vi "Custom Device CORE.vi"(8 "error in (no error)":errorcluster, 11 "CDW_MetaDataObj":refnum<class "NIVS_Consolidated_CDW_MetaDataObj.lvclass">) -> (0 "error out":errorcluster)   [LabVIEW 2019, in "NIVS_Consolidated_CDW_MetaDataObj.lvclass"]
doc: "This VI is the Core VI for the Custom Device Wizard.\n\nWritten by:\nStephan Daunke\n\nDate:\n2014/01/27\n\nCompany:\nNational Instruments Germany GmbH"
uses:
  NIVS_Consolidated_CDW_MetaDataObj.lvclass
  Action.ctl
  CD Shared lvlib.vi
  CD Shared lvlib.ctl
  CD System Explorer lvlib.vi
  CD System Explorer lvlib.ctl
  Common.ctl
  Utility folder.vi
  Utility folder.ctl
  CD Engine lvlib.vi
  CD Engine lvlib.ctl
  Common.vi
  Add Item - Type.ctl
  Build Spec System Explorer.ctl
  Build Spec Engine.vi
  Build Spec Engine.ctl
  <vilib>/Utility/config.llb/NI_LVConfig.lvlib
  <vilib>/Utility/config.llb/Write Key (String).vi
  <vilib>/Utility/traverseref.llb/TRef TravTarget.ctl
  <vilib>/Utility/Data Type/NI_Data Type.lvlib
  Internal data.ctl
  Template Classes/NIVS_CD Template/NIVS_CD Template.lvclass
  Template Classes/NIVS_PPLCD Template/NIVS_PPLCD Template.lvclass
  Build Spec System Explorer.vi
  <vilib>/Utility/config.llb/Write Key (Path).vi
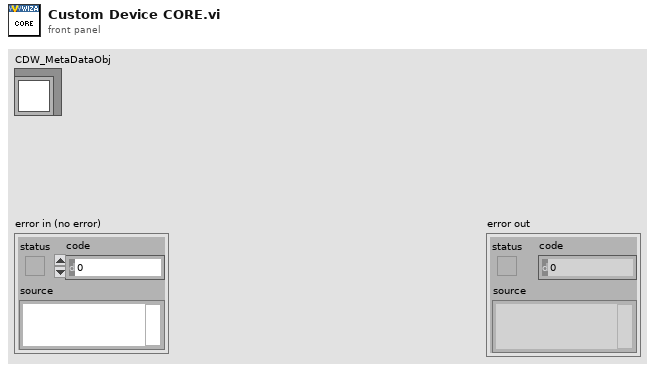
[diagram p1: front panel]
types:
  T1 = typedef "NIVS_Consolidated_CDW_MetaDataObj.lvclass/Internal data.ctl" = cluster{"CD GUID":string, "Extra Page GUIDs":string[], "System Explorer Library":refnum<vi>, "Shared Library":refnum<vi>, "Engine Library":refnum<vi>}
  T2 = typedef "NIVS_Consolidated_CDW_MetaDataObj.lvclass/Action.ctl" = enum16{"Project - Create Custom Device folder", "PC - Create GUID for each extra page", "PC-Utility - Create folder and copy -Copy .LLB to NI VeriStand dir-", "PC-Utility - Change -Copy .LLB to NI VeriStand dir-", "PC-Shared - Create folder and copy Constants.vi", "PC-Shared - Change Constants.vi content", "PC-Shared - Create library", "PC-Shared - Add folders and VIs to library", "PC-System Explorer - Create folder and copy templates", "PC-System Explorer - Create extra pages", "PC-System Explorer - Create library", "PC-System Explorer - Add folders and VIs to library", "PC-Engine - Create folder and copy the RT Template", "PC-Engine - Create library", "PC-Engine - Add virtual folders and VIs to library", "PC-XML - Create and change file", "PC-Help - Copy HTML Files", "Project - Read project file content", "Project - Edit Utility section", "Project - Edit XML section", "Project - Edit Engine Library section", "Project - Edit Shared Library section", "Project - Edit System Explorer Library section", "Project - Edit Custom Device Name", "Project - Edit System Explorer LLB Name", "Project - Edit Engine LLB OS dependent file name", "Project - Copy Configuration file", "Project - Write new project file"}
  T3 = typedef "NIVS_Consolidated_CDW_MetaDataObj.lvclass/Utility folder.ctl" = enum16{"Utility.FolderName", "Utility.PPL Tools Folder Path", "Utility.Copy .llb to NI VeriStand dir.FileName", "Utility.Copy .llb to NI VeriStand dir.FilePathAndName", "Utility.LLB Pre Build.FilePathAndName"}
  T4 = typedef "NIVS_Consolidated_CDW_MetaDataObj.lvclass/CD Shared lvlib.ctl" = enum16{"LibraryFileName", "LibraryFolderName", "ConstantsVI.VIPathAndName", "Shared.FolderName", "Shared.Types.FolderName", "Shared.Constants.VIName", "Shared.Constants.VITemplateName", "Shared.Constants.VITemplatePathAndName", "Shared.CompiledSettings.RelativePath", "Shared.Constants.RelativePath", "Shared.CompiledSettings.Name", "Shared.CompiledSettings.Name.NoExtension", "Shared.CompiledSettings.ClusterName"}
  T5 = typedef "NIVS_Consolidated_CDW_MetaDataObj.lvclass/Common.ctl" = enum16{"ProjectName", "TemplatesFolderName", "PPLTemplatesFolderName", "ProjectTemplatePathAndName", "TimingAndSyncFolderName", "CustomDeviceFolderName", "PathToTemplates", "PathToConfigurationFile", "ProjectConfigurationName"}
  T6 = typedef "NIVS_Consolidated_CDW_MetaDataObj.lvclass/Add Item - Type.ctl" = string
  T7 = typedef "NIVS_Consolidated_CDW_MetaDataObj.lvclass/CD System Explorer lvlib.ctl" = enum16{"LibraryFileName", "LibraryFolderName", "System Explorer.FolderName", "System Explorer.Dynamically Called.FolderName", "System Explorer.Dynamically Called.Extra Pages.FolderName", "System Explorer.Dynamically Called.Extra Pages.TemplatePathAndName", "System Explorer.Dynamically Called.Main Page.VIName", "System Explorer.Dynamically Called.Main Page.TemplatePathAndName", "System Explorer.Dynamically Called.Initialization VI.VIName", "System Explorer.Dynamically Called.Initialization VI.TemplatePathAndName", "System Explorer.SubVI.FolderName", "System Explorer.Types.FolderName", "System Explorer.ActionVIOnCompile.VIName", "System Explorer.ExportConfigRTM.VIName", "System Explorer.LoadHelpFile.VIName"}
  T8 = typedef "TRef TravTarget.ctl" = enum16{"FP", "BD", "Other"}
  T9 = typedef "NIVS_Consolidated_CDW_MetaDataObj.lvclass/CD Engine lvlib.ctl" = enum16{"LibraryFileName", "LibraryFolderName", "Engine.FolderName", "Engine.Init.FolderName", "Engine.Run.FolderName", "Engine.Shutdown.FolderName", "Types.FolderName", "Engine.RT Driver VI.TemplatePath", "Engine.RT Driver VI.FileName", "Engine.RTStateVariables.Name", "Engine.RTStateVariables.Name.NoExtension", "Engine.Async.NameExtension", "Engine.Async.TemplateName"}
  T10 = typedef "NIVS_Consolidated_CDW_MetaDataObj.lvclass/Build Spec System Explorer.ctl" = enum16{"Destinations.LLBFileName"}
  T11 = typedef "NIVS_Consolidated_CDW_MetaDataObj.lvclass/Build Spec Engine.ctl" = enum16{"Destinations.LLBWindowsFileName", "Destinations.LLBVxWorksFileName", "Destinations.LLBPharlapFileName", "Destinations.LLBLinuxARMFileName", "Destinations.LLBLinux64FileName"}
  T12 = enum16{"open", "replace", "create", "open or create", "replace or create", "replace or create with confirmation"}
  T13 = typedef "NI_LVConfig.lvlib/Config Data RefNum.ctl" = refnum<k1>
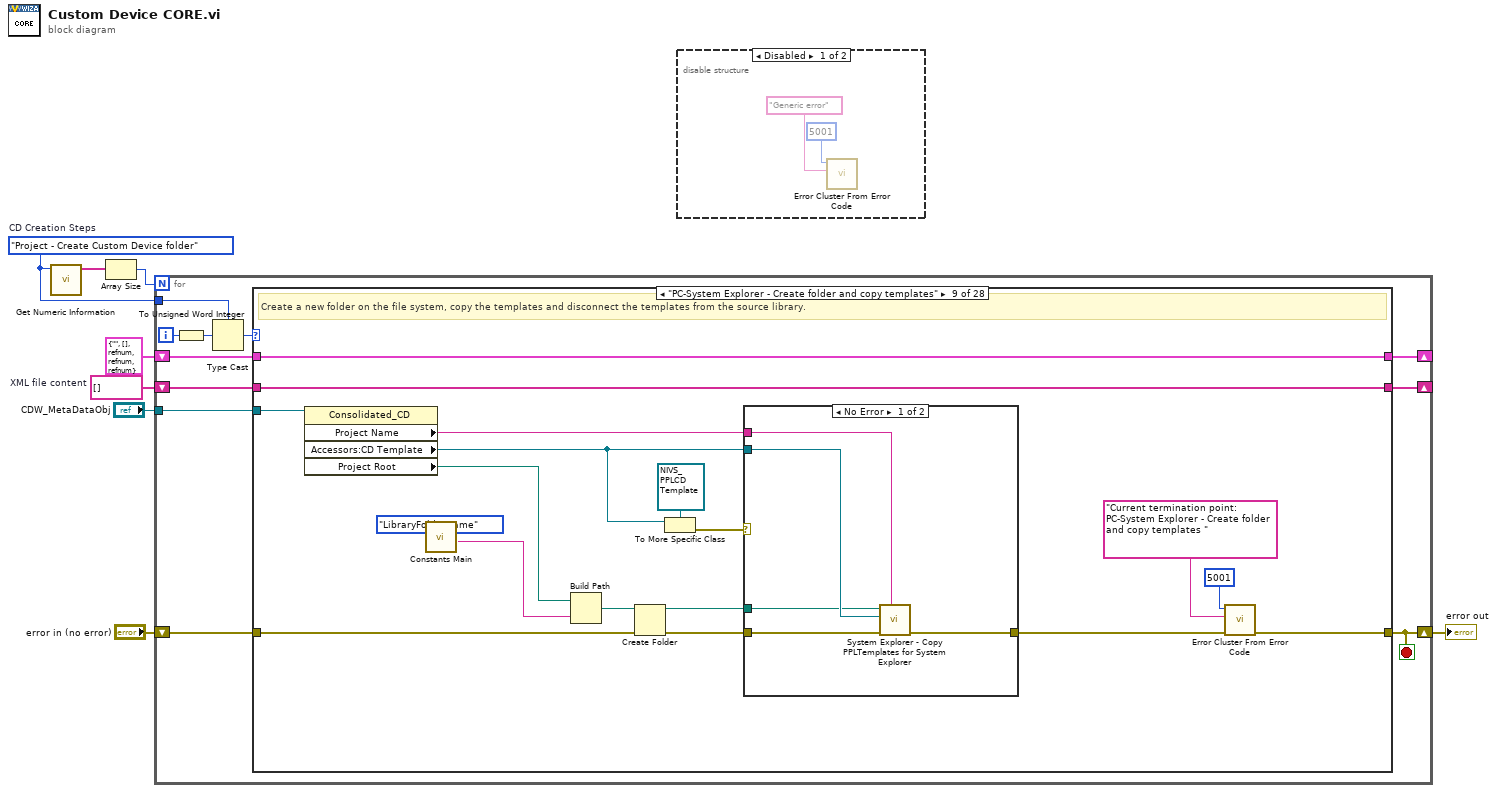
[diagram p0: block diagram]
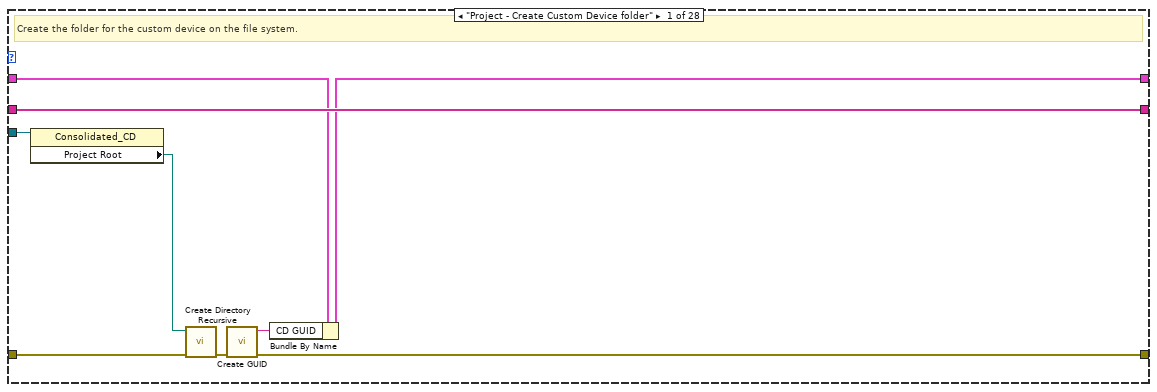
[diagram p3: hidden frame]
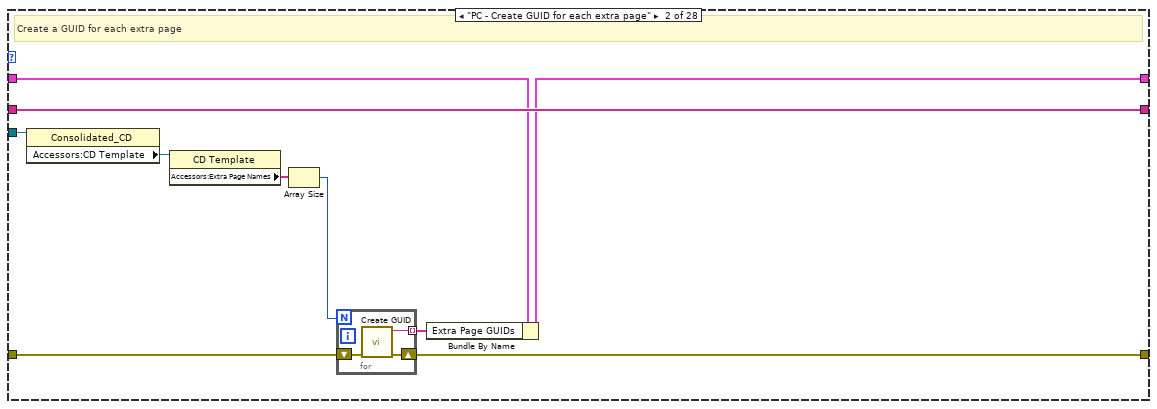
[diagram p4: hidden frame]
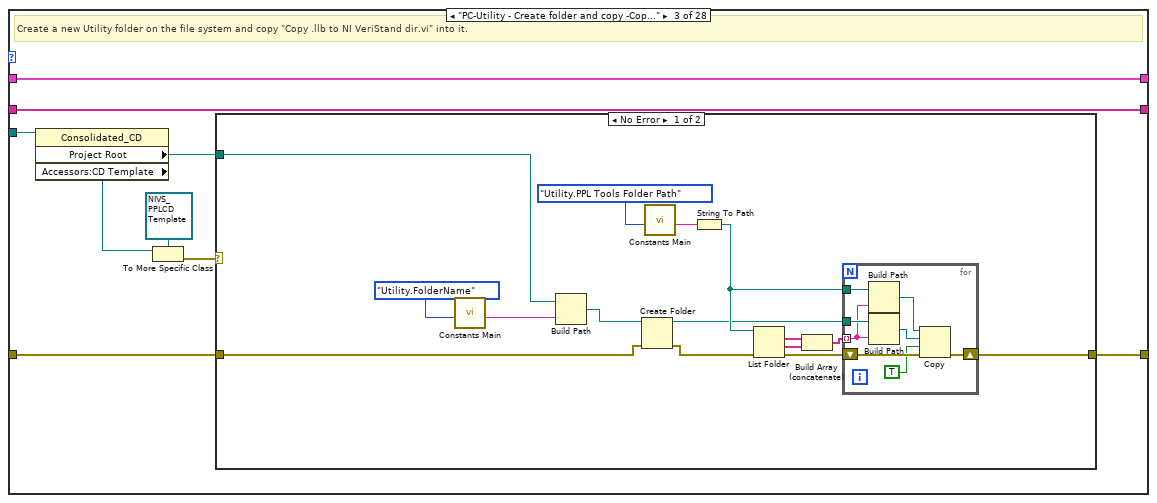
[diagram p5: hidden frame]
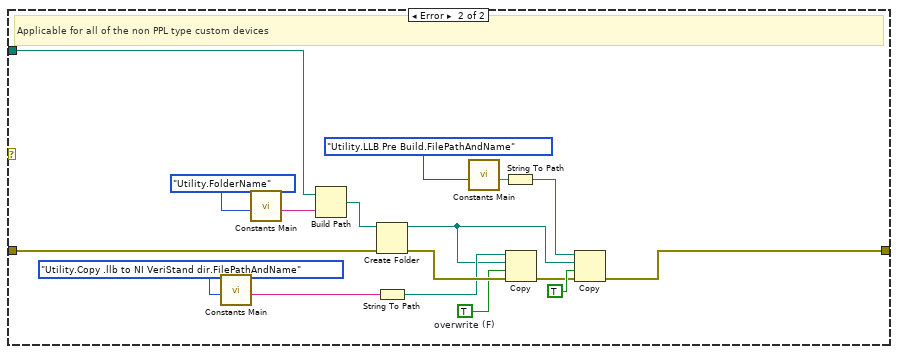
[diagram p6: hidden frame]
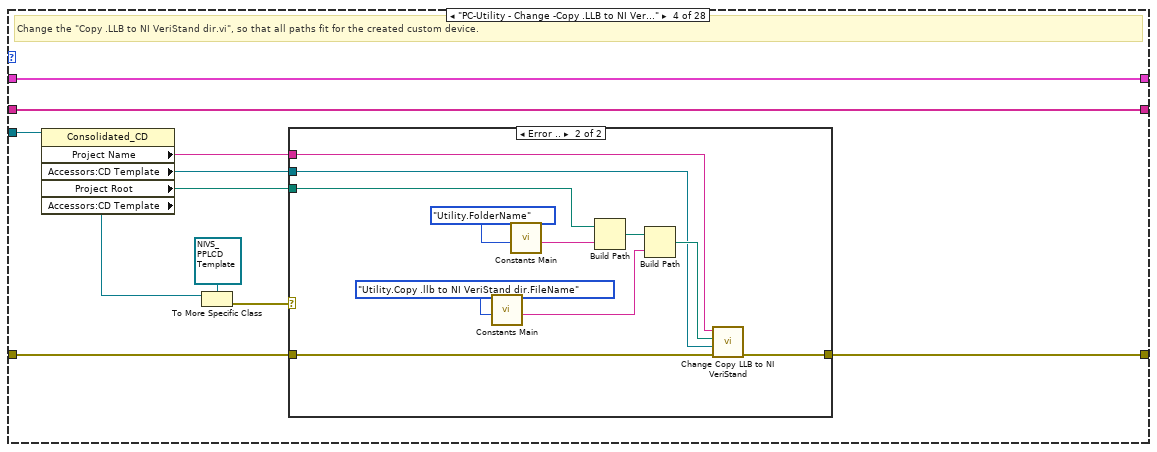
[diagram p7: hidden frame]
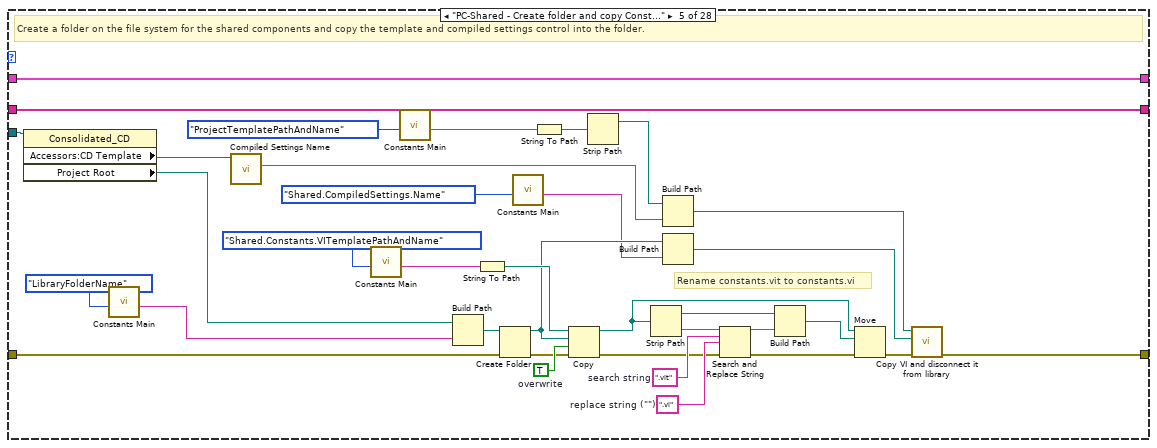
[diagram p9: hidden frame]
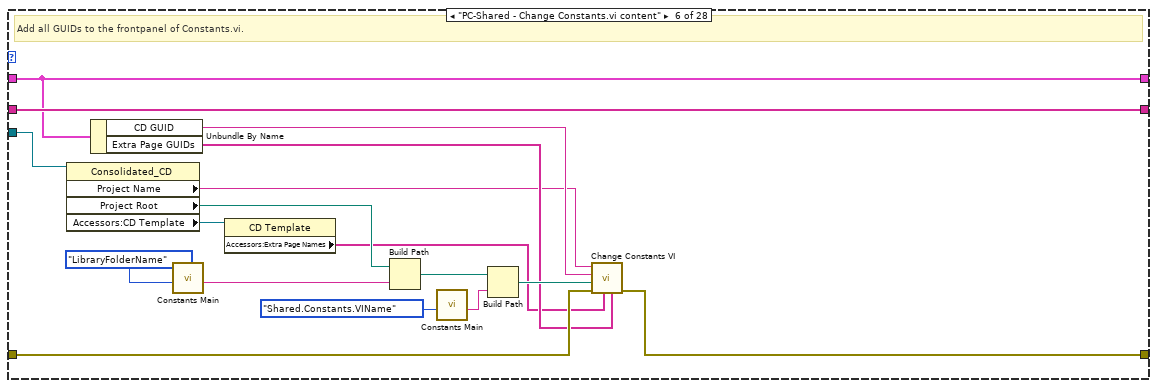
[diagram p10: hidden frame]
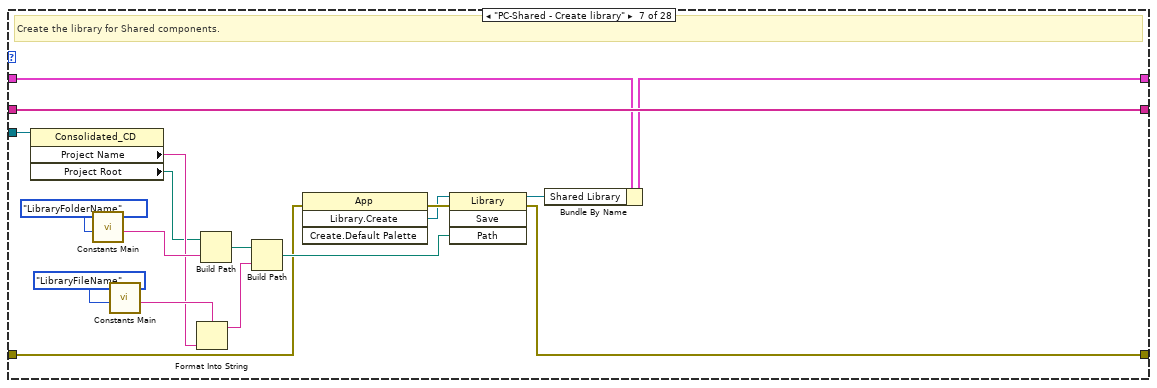
[diagram p11: hidden frame]
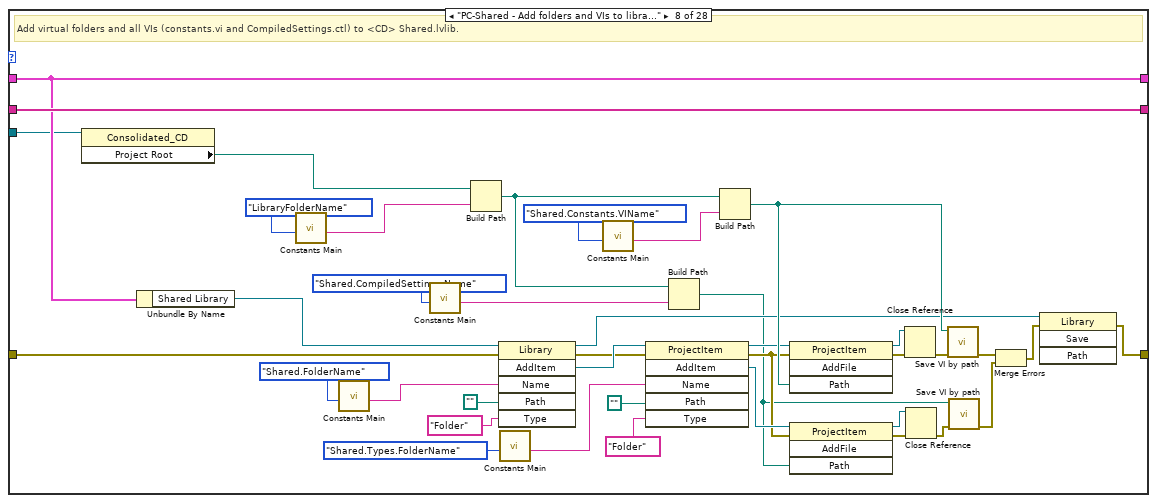
[diagram p12: hidden frame]
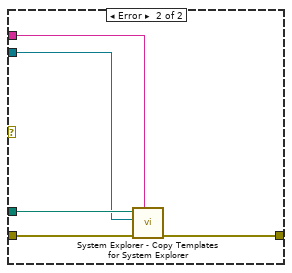
[diagram p13: hidden frame]
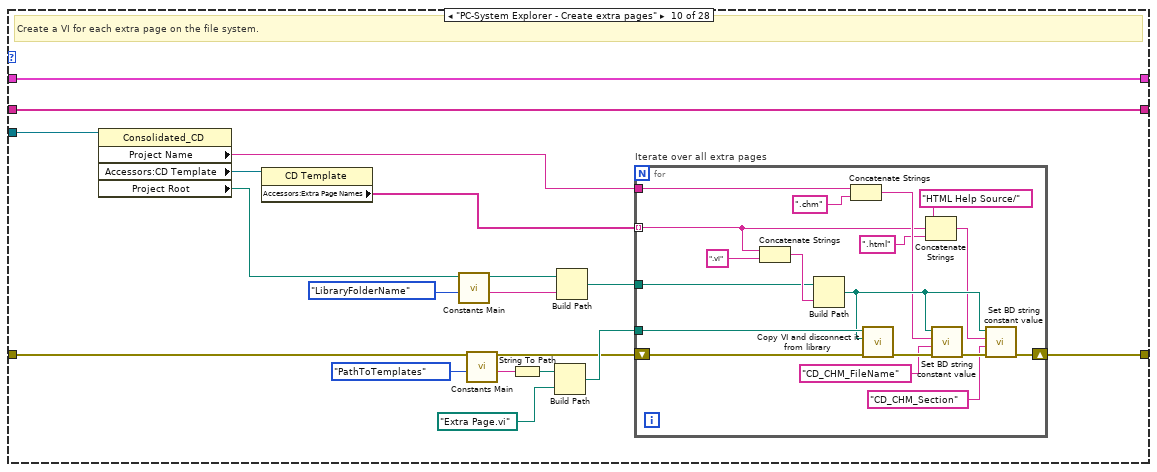
[diagram p14: hidden frame]
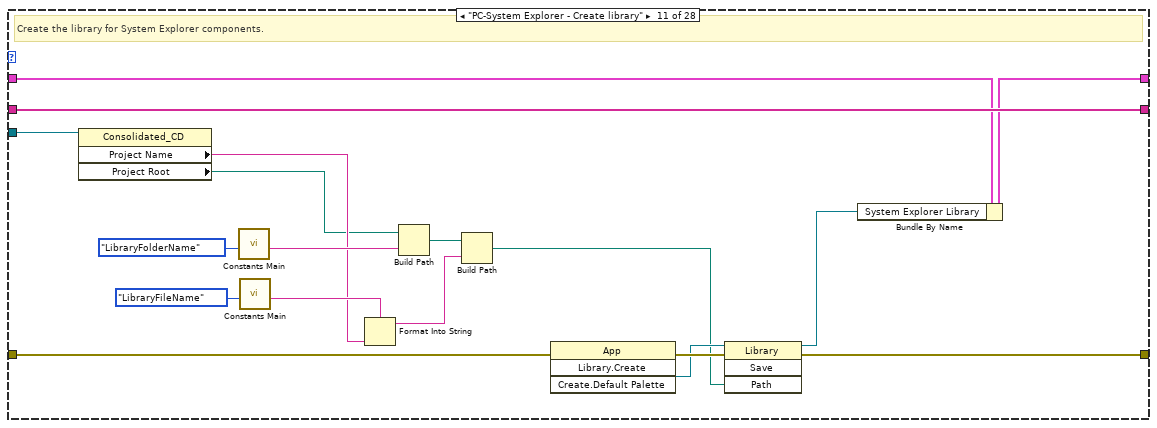
[diagram p15: hidden frame]
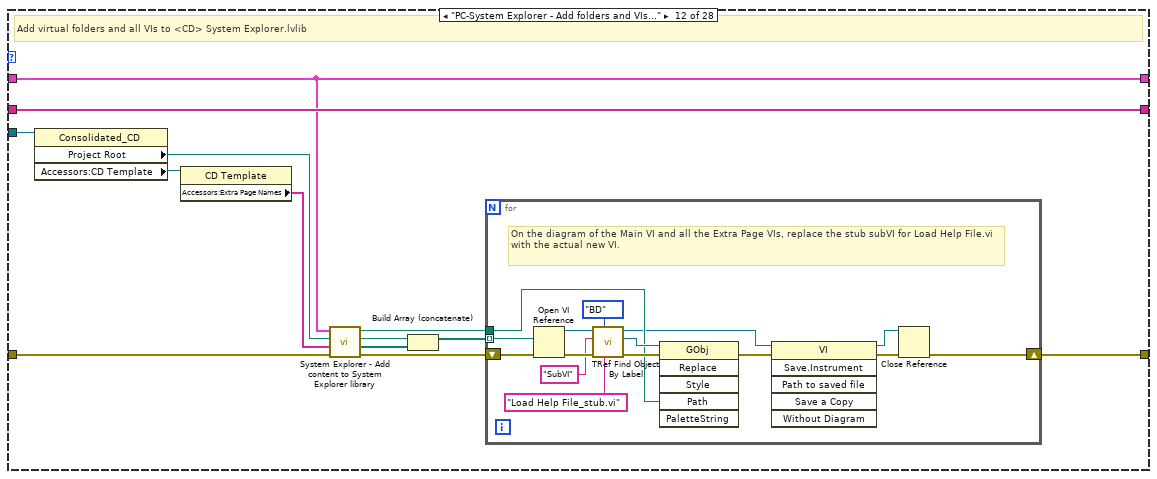
[diagram p16: hidden frame]
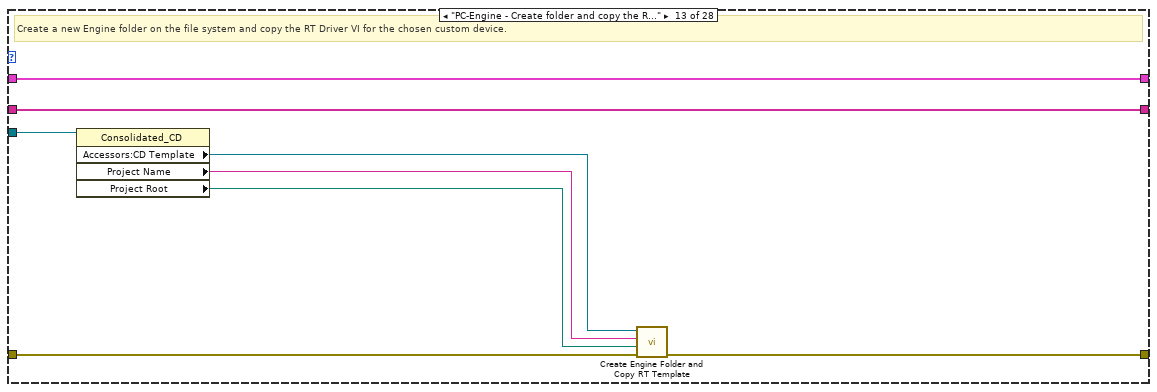
[diagram p17: hidden frame]
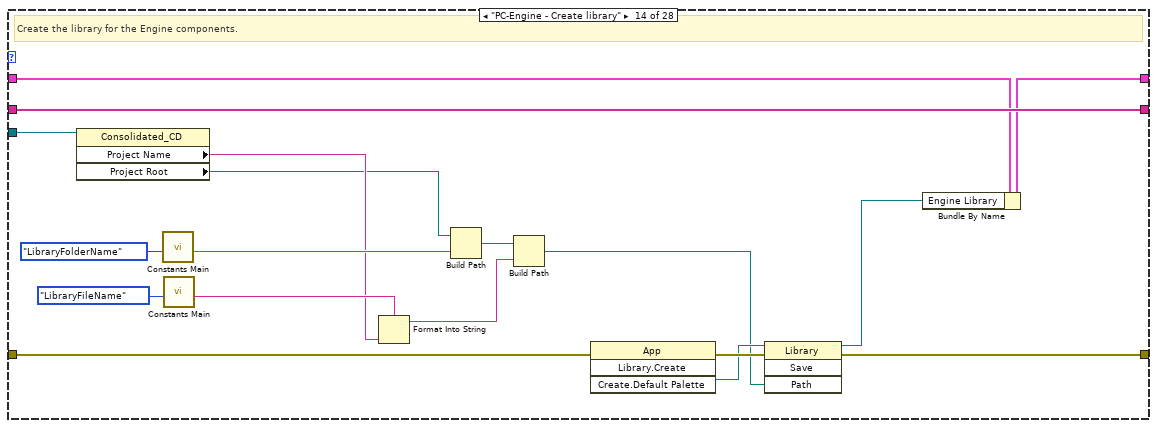
[diagram p18: hidden frame]
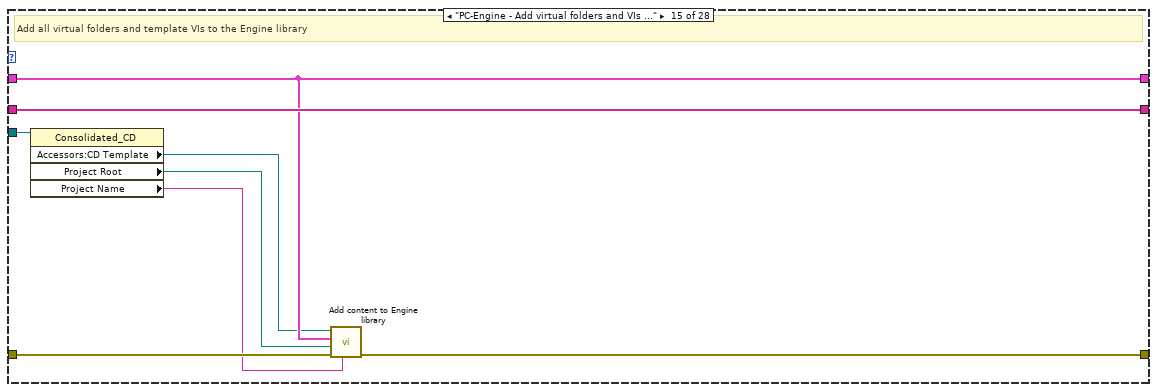
[diagram p19: hidden frame]
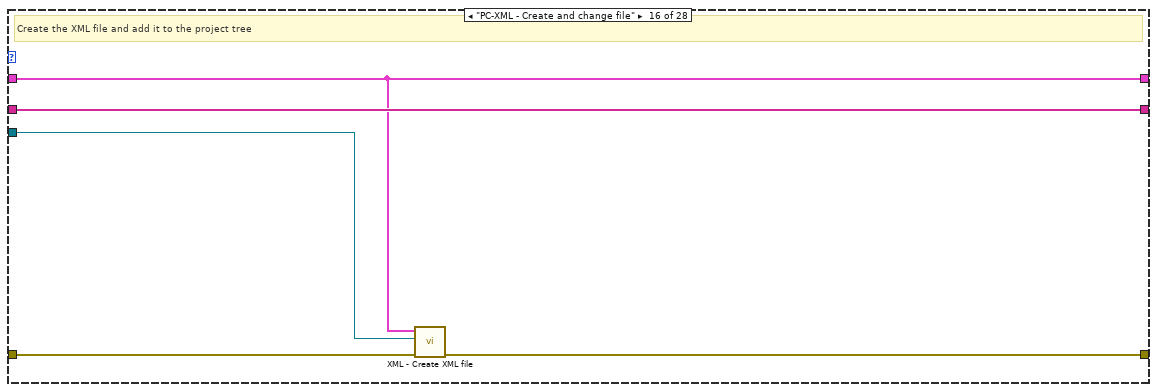
[diagram p20: hidden frame]
diagram:
  w4 = Action."Project - Create Custom Device folder"  # CD Creation Steps
  w5 = string[] []  # XML file content
  n1 = call <vilib>:"Get Numeric Information.vi"("variant"=w4) -> ("enum names"=w3:string[])  [unwired: 7 in, 3 out]
  n2 = Array Size(array=w3) -> (size(s)=w2:i32)
  n3 = for {
    N: w2 -> [_]
    shift-right: [w16] -> _
    shift-left: T1 {"CD GUID"="", "Extra Page GUIDs"=[], "System Explorer Library"=refnum, "Shared Library"=refnum, "Engine Library"=refnum} ("CD Wizard - Internal Data") -> [w18]
    shift-right: [w15] -> _
    shift-left: w5 -> [w17]
    shift-right: [w14] -> w6
    shift-left: "error in (no error)" -> [w19]
    tunnel: w4 -> [w12]
    tunnel: "CDW_MetaDataObj" -> [w11]
    i -> [w13]
    stop <- w14 stop-if-true
    n4 = To Unsigned Word Integer(number=w13) -> (unsigned 16bit integer=w9:u16)
    n5 = Type Cast(type=w12, x=w9) -> (*(type *) &x=w10:T2)
    n6 = case shown="\"PC-System Explorer - Create folder and copy templates\"" w10 {
      tunnel: w19 -> [w24 w37 w46 w96 w118 w158 w169 w186 w231 w256 w289 w315 w338 w343 w364 w369 w387 w417 w430 w462 w481 w485 w515 w549 w560 w578 w615 w631]
      tunnel: [w25 w36 w49 w100 w120 w164 w170 w184 w223 w266 w290 w310 w337 w346 w363 w368 w386 w423 w439 w467 w480 w495 w519 w548 w567 w590 w614 w638] -> w14
      tunnel: w18 -> [w22 w34 w48 w99 w119 w155 w173 w204 w234 w265 w295 w313 w336 w350 w361 w367 w382 w429 w442 w464 w479 w486 w516 w545 w564 w596 w627 w663]
      tunnel: w17 -> [w28 w38 w50 w101 w148 w165 w183 w222 w240 w267 w303 w316 w339 w357 w365 w370 w409 _ w441 w466 w478 w490 w517 w546 w562 w591 w626 w657]
      tunnel: [w27 w33 w48 w99 w119 w155 w172 w204 w234 w265 w296 w313 w336 w349 w361 w367 w382 w429 w442 w464 w479 w486 w516 w545 w564 w596 w627 w663] -> w16
      tunnel: [w28 w38 w50 w101 w148 w165 w183 w222 w240 w267 w303 w316 w339 w357 w365 w370 w409 w422 w440 w465 w482 w496 w518 w547 w561 w579 w626 w657] -> w15
      tunnel: w11 -> [w21 w32 w45 w98 w117 w157 w168 w188 w233 w255 w288 w309 w335 w342 w362 w366 w376 _ _ w461 w477 w484 w514 w544 w559 w577 w620 w630]
      frame "Project - Create Custom Device folder" {
        # "Create the folder for the custom device on the file system."
        n7 = property class="Consolidated_CD"(reference=w21) -> ("Project Root"=w20:path)  [unwired: 1 in, 2 out]
        n8 = call <vilib>:"Create Directory Recursive.vi"("error in (no error)"=w24, "directory"=w20) -> ("error out"=w23:errorcluster)  [unwired: 3 in, 2 out]
        n9 = call "Create GUID.vi"("error in (no error)"=w23) -> ("error out"=w25:errorcluster, "Generated GUID"=w26:string)  [unwired: 9 in]
        n10 = Bundle By Name(cluster=w22, "CD GUID"=w26) -> (w27:T1)
      }
      frame "PC - Create GUID for each extra page" {
        # "Create a GUID for each extra page"
        n11 = property class="Consolidated_CD"(reference=w32) -> ("Accessors:CD Template"=w31:refnum<class "NIVS_CD Template.lvclass">)  [unwired: 1 in, 2 out]
        n12 = property class="CD Template"(reference=w31) -> ("Accessors:Extra Page Names"=w30:string[])  [unwired: 1 in, 2 out]
        n13 = Array Size(array=w30) -> (size(s)=w29:i32)
        n14 = for {
          N: w29 -> [_]
          shift-right: [w40] -> w36
          shift-left: w37 -> [w41]
          tunnel: [w39] -> w35 mode=indexing
          n15 = call "Create GUID.vi"("error in (no error)"=w41) -> ("error out"=w40:errorcluster, "Generated GUID"=w39:string)  [unwired: 9 in]
        }
        n16 = Bundle By Name(cluster=w34, "Extra Page GUIDs"=w35) -> (w33:T1)
      }
      frame "PC-Utility - Create folder and copy -Copy .LLB to NI VeriStand dir-" {
        # "Create a new Utility folder on the file system and copy \"Copy .llb to NI VeriStand dir.vi\" into it."
        n17 = property class="Consolidated_CD"(reference=w45) -> ("Project Root"=w47:path, "Accessors:CD Template"=w42:refnum<class "NIVS_CD Template.lvclass">)  [unwired: 1 in, 2 out]
        n18 = To More Specific Class(target class=refnum<class "NIVS_PPLCD Template.lvclass"> refnum ("NIVS_PPLCD Template.lvclass"), reference=w42) -> (error out=w43:errorcluster)  [unwired: 1 in, 1 out]
        n19 = case shown="No Error" w43 {
          tunnel: [w51 w77] -> w49
          tunnel: w47 -> [w59 w76]
          tunnel: w46 -> [w60 w75]
          frame No Error {
            n20 = call-poly "Constants Main.vi"("Action"=Utility_folder."Utility.FolderName") -> ("Output"=w61:string)  [unwired: 10 in]
            n21 = Build Path(base path=w59, name or relative path=w61) -> (appended path=w65:path)
            n22 = Create Folder(path (use dialog)=w65, error in=w60) -> (created path=w56:path, error out=w55:errorcluster)  [unwired: 1 in, 1 out]
            n23 = call-poly "Constants Main.vi"("Action"=Utility_folder."Utility.PPL Tools Folder Path") -> ("Output"=w63:string)  [unwired: 10 in]
            n24 = String To Path(string=w63) -> (path=w57:path)
            n25 = List Folder(path=w57, error in=w55) -> (filenames=w54:string[], folder names=w53:string[], error out=w58:errorcluster)  [unwired: 2 in, 1 out]
            n26 = Build Array (concatenate)(w54, w53) -> (w52:string[])
            n27 = for {
              tunnel: w52 -> [w68] mode=indexing
              tunnel: w57 -> [w71]
              shift-right: [w72] -> w51
              shift-left: w58 -> [w73]
              tunnel: w56 -> [w69]
              n28 = Build Path(base path=w71, name or relative path=w68) -> (appended path=w70:path)
              n29 = Build Path(base path=w69, name or relative path=w68) -> (appended path=w67:path)
              n30 = Copy(8:w73, 9:TRUE ("overwrite (F)"), 10:w67, 11:w70) -> (0:w72:errorcluster)  [unwired: 1 in, 2 out]
            }
          }
          frame Error {
            w88 = TRUE  # overwrite (F)
            # "Applicable for all of the non PPL type custom devices"
            n31 = call-poly "Constants Main.vi"("Action"=Utility_folder."Utility.Copy .llb to NI VeriStand dir.FilePathAndName") -> ("Output"=w86:string)  [unwired: 10 in]
            n32 = call-poly "Constants Main.vi"("Action"=Utility_folder."Utility.FolderName") -> ("Output"=w83:string)  [unwired: 10 in]
            n33 = Build Path(base path=w76, name or relative path=w83) -> (appended path=w90:path)
            n34 = Create Folder(path (use dialog)=w90, error in=w75) -> (created path=w82:path, error out=w89:errorcluster)  [unwired: 1 in, 1 out]
            n35 = String To Path(string=w86) -> (path=w85:path)
            n36 = call-poly "Constants Main.vi"("Action"=Utility_folder."Utility.LLB Pre Build.FilePathAndName") -> ("Output"=w80:string)  [unwired: 10 in]
            n37 = String To Path(string=w80) -> (path=w79:path)
            n38 = Copy(8:w89, 9:w88, 10:w82, 11:w85) -> (0:w74:errorcluster)  [unwired: 3 out]
            n39 = Copy(8:w74, 9:TRUE ("overwrite (F)"), 10:w82, 11:w79) -> (0:w77:errorcluster)  [unwired: 3 out]
          }
        }
      }
      frame "PC-Utility - Change -Copy .LLB to NI VeriStand dir-" {
        # "Change the \"Copy .LLB to NI VeriStand dir.vi\", so that all paths fit for the created custom device."
        n40 = property class="Consolidated_CD"(reference=w98) -> ("Project Name"=w97:string, "Accessors:CD Template"=w93:refnum<class "NIVS_CD Template.lvclass">, "Project Root"=w95:path, "Accessors:CD Template"=w92:refnum<class "NIVS_CD Template.lvclass">)  [unwired: 1 in, 2 out]
        n41 = To More Specific Class(target class=refnum<class "NIVS_PPLCD Template.lvclass"> refnum ("NIVS_PPLCD Template.lvclass"), reference=w92) -> (error out=w91:errorcluster)  [unwired: 1 in, 1 out]
        n42 = case shown="Error .." w91 {
          tunnel: [w102 w108] -> w100
          tunnel: w97 -> [_ w106]
          tunnel: w96 -> [w102 w105]
          tunnel: w95 -> [_ w104]
          tunnel: w93 -> [_ w103]
          frame No Error {
            # "No need to do this for the PPL based CDs"
          }
          frame Error {
            n43 = call-poly "Constants Main.vi"("Action"=Utility_folder."Utility.Copy .llb to NI VeriStand dir.FileName") -> ("Output"=w109:string)  [unwired: 10 in]
            n44 = call-poly "Constants Main.vi"("Action"=Utility_folder."Utility.FolderName") -> ("Output"=w111:string)  [unwired: 10 in]
            n45 = Build Path(base path=w104, name or relative path=w111) -> (appended path=w110:path)
            n46 = Build Path(base path=w110, name or relative path=w109) -> (appended path=w107:path)
            n47 = call "Change Copy LLB to NI VeriStand.vi"("error in (no error)"=w105, "CD Template"=w103, "Copy .LLB to ... path"=w107, "CD Name"=w106) -> ("error out"=w108:errorcluster)  [unwired: 7 in]
          }
        }
      }
      frame "PC-Shared - Create folder and copy Constants.vi" {
        w137 = ".vi"  # replace string ("")
        w138 = ".vit"  # search string
        w142 = TRUE  # overwrite
        # "Rename constants.vit to constants.vi"
        # "Create a folder on the file system for the shared components and copy the template and compiled settings control into the folder."
        n48 = property class="Consolidated_CD"(reference=w117) -> ("Accessors:CD Template"=w115:refnum<class "NIVS_CD Template.lvclass">, "Project Root"=w116:path)  [unwired: 1 in, 2 out]
        n49 = call-poly "Constants Main.vi"("Action"=CD_Shared_lvlib."LibraryFolderName") -> ("Output"=w145:string)  [unwired: 10 in]
        n50 = call-dynamic "Compiled Settings Name.vi"("CD Template in"=w115) -> ("Compiled Settings Name"=w114:string)  [unwired: 10 in]
        n51 = call-poly "Constants Main.vi"("Action"=CD_Shared_lvlib."Shared.Constants.VITemplatePathAndName") -> ("Output"=w143:string)  [unwired: 10 in]
        n52 = call-poly "Constants Main.vi"("Action"=Common."ProjectTemplatePathAndName") -> ("Output"=w129:string)  [unwired: 10 in]
        n53 = Build Path(base path=w116, name or relative path=w145) -> (appended path=w147:path)
        n54 = String To Path(string=w143) -> (path=w135:path)
        n55 = Create Folder(path (use dialog)=w147, error in=w118) -> (created path=w126:path, error out=w136:errorcluster)  [unwired: 1 in, 1 out]
        n56 = call-poly "Constants Main.vi"("Action"=CD_Shared_lvlib."Shared.CompiledSettings.Name") -> ("Output"=w121:string)  [unwired: 10 in]
        n57 = String To Path(string=w129) -> (path=w128:path)
        n58 = Copy(8:w136, 9:w142, 10:w126, 11:w135) -> (0:w134:errorcluster, 3:w131:path)  [unwired: 2 out]
        n59 = Strip Path(path=w128) -> (stripped path=w127:path)  [unwired: 1 out]
        n60 = Strip Path(path=w131) -> (stripped path=w141:path, name=w140:string)
        n61 = Build Path(base path=w127, name or relative path=w114) -> (appended path=w125:path)
        n62 = Build Path(base path=w126, name or relative path=w121) -> (appended path=w124:path)
        n63 = Search and Replace String(input string=w140, search string=w138, replace string=w137, error in=w134) -> (result string=w139:string, error out=w133:errorcluster)  [unwired: 4 in, 2 out]
        n64 = Build Path(base path=w141, name or relative path=w139) -> (appended path=w132:path)
        n65 = Move(source path=w131, error in=w133, 10:w132) -> (error out=w123:errorcluster)  [unwired: 2 in, 2 out]
        n66 = call "Copy VI and disconnect it from library.vi"("error in (no error)"=w123, "VI Target Path"=w124, "VI Source Path"=w125) -> ("error out"=w120:errorcluster)  [unwired: 8 in]
      }
      frame "PC-Shared - Change Constants.vi content" {
        # "Add all GUIDs to the frontpanel of Constants.vi."
        n67 = property class="Consolidated_CD"(reference=w157) -> ("Project Name"=w151:string, "Project Root"=w156:path, "Accessors:CD Template"=w150:refnum<class "NIVS_CD Template.lvclass">)  [unwired: 1 in, 2 out]
        n68 = Unbundle By Name(w155) -> ("CD GUID"=w153:string, "Extra Page GUIDs"=w152:string[])
        n69 = call-poly "Constants Main.vi"("Action"=CD_Shared_lvlib."LibraryFolderName") -> ("Output"=w159:string)  [unwired: 10 in]
        n70 = property class="CD Template"(reference=w150) -> ("Accessors:Extra Page Names"=w149:string[])  [unwired: 1 in, 2 out]
        n71 = Build Path(base path=w156, name or relative path=w159) -> (appended path=w163:path)
        n72 = call-poly "Constants Main.vi"("Action"=CD_Shared_lvlib."Shared.Constants.VIName") -> ("Output"=w161:string)  [unwired: 10 in]
        n73 = Build Path(base path=w163, name or relative path=w161) -> (appended path=w154:path)
        n74 = call "Change Constants VI.vi"("Extra Page GUIDs"=w152, "Extra Page Names"=w149, "error in (no error)"=w158, "Constants.vi path"=w154, "CD GUID"=w153, "CD Name"=w151) -> ("error out"=w164:errorcluster)  [unwired: 5 in]
      }
      frame "PC-Shared - Create library" {
        # "Create the library for Shared components."
        n75 = property class="Consolidated_CD"(reference=w168) -> ("Project Name"=w167:string, "Project Root"=w166:path)  [unwired: 1 in, 2 out]
        n76 = call-poly "Constants Main.vi"("Action"=CD_Shared_lvlib."LibraryFolderName") -> ("Output"=w177:string)  [unwired: 10 in]
        n77 = call-poly "Constants Main.vi"("Action"=CD_Shared_lvlib."LibraryFileName") -> ("Output"=w178:string)  [unwired: 10 in]
        n78 = Format Into String(format string=w178, w167) -> (resulting string=w181:string)  [unwired: 2 in, 1 out]
        n79 = Build Path(base path=w166, name or relative path=w177) -> (appended path=w182:path)
        n80 = Build Path(base path=w182, name or relative path=w181) -> (appended path=w174:path)
        n81 = invoke class="App" method="Library.Create"(error in=w169) -> (error out=w176:errorcluster, "Create Library"=w175:refnum<vi>)  [unwired: 3 in, 2 out]
        n82 = invoke class="Library" method="Save"(reference=w175, error in=w176, "Path"=w174) -> (reference out=w171:refnum<vi>, error out=w170:errorcluster)  [unwired: 1 in, 2 out]
        n83 = Bundle By Name(cluster=w173, "Shared Library"=w171) -> (w172:T1)
      }
      frame "PC-Shared - Add folders and VIs to library" {
        # "Add virtual folders and all VIs (constants.vi and CompiledSettings.ctl) to <CD> Shared.lvlib."
        n84 = property class="Consolidated_CD"(reference=w188) -> ("Project Root"=w187:path)  [unwired: 1 in, 2 out]
        n85 = Unbundle By Name(w204) -> ("Shared Library"=w206:refnum<vi>)
        n86 = call-poly "Constants Main.vi"("Action"=CD_Shared_lvlib."LibraryFolderName") -> ("Output"=w201:string)  [unwired: 10 in]
        n87 = call-poly "Constants Main.vi"("Action"=CD_Shared_lvlib."Shared.FolderName") -> ("Output"=w202:string)  [unwired: 10 in]
        n88 = call-poly "Constants Main.vi"("Action"=CD_Shared_lvlib."Shared.CompiledSettings.Name") -> ("Output"=w193:string)  [unwired: 10 in]
        n89 = Build Path(base path=w187, name or relative path=w201) -> (appended path=w198:path)
        n90 = invoke class="Library" method="AddItem"(reference=w206, error in=w186, "Name"=w202, "Path"=path "", "Type"=T6 "Folder" ("Add Item - Type")) -> (reference out=w212:refnum<vi>, error out=w207:errorcluster, "AddItem"=w209:refnum<vi>)  [unwired: 1 in, 3 out]
        n91 = call-poly "Constants Main.vi"("Action"=CD_Shared_lvlib."Shared.Types.FolderName") -> ("Output"=w220:string)  [unwired: 10 in]
        n92 = call-poly "Constants Main.vi"("Action"=CD_Shared_lvlib."Shared.Constants.VIName") -> ("Output"=w189:string)  [unwired: 10 in]
        n93 = invoke class="ProjectItem" method="AddItem"(reference=w209, error in=w207, "Name"=w220, "Path"=path "", "Type"=T6 "Folder" ("Add Item - Type")) -> (reference out=w211:refnum<vi>, error out=w199:errorcluster, "AddItem"=w200:refnum<vi>)  [unwired: 1 in, 3 out]
        n94 = Build Path(base path=w198, name or relative path=w193) -> (appended path=w197:path)
        n95 = Build Path(base path=w198, name or relative path=w189) -> (appended path=w213:path)
        n96 = invoke class="ProjectItem" method="AddFile"(reference=w211, error in=w199, "Path"=w213) -> (reference out=w216:refnum<vi>, error out=w215:errorcluster)  [unwired: 1 in, 2 out]
        n97 = invoke class="ProjectItem" method="AddFile"(reference=w200, error in=w199, "Path"=w197) -> (reference out=w191:refnum<vi>, error out=w190:errorcluster)  [unwired: 1 in, 2 out]
        n98 = Close Reference(reference=w216, error in (no error)=w215) -> (error out=w217:errorcluster)
        n99 = Close Reference(reference=w191, error in (no error)=w190) -> (error out=w192:errorcluster)
        n100 = call "Save VI by path.vi"("error in (no error)"=w217, "VI path"=w213) -> ("error out"=w214:errorcluster)  [unwired: 9 in]
        n101 = call "Save VI by path.vi"("error in (no error)"=w192, "VI path"=w197) -> ("error out"=w195:errorcluster)  [unwired: 9 in]
        n102 = Merge Errors(w214, w195) -> (w196:errorcluster)
        n103 = invoke class="Library" method="Save"(reference=w212, error in=w196) -> (error out=w184:errorcluster)  [unwired: 2 in, 3 out]
      }
      frame "PC-System Explorer - Create folder and copy templates" {
        # "Create a new folder on the file system, copy the templates and disconnect the templates from the source library."
        n104 = property class="Consolidated_CD"(reference=w233) -> ("Project Name"=w232:string, "Accessors:CD Template"=w229:refnum<class "NIVS_CD Template.lvclass">, "Project Root"=w230:path)  [unwired: 1 in, 2 out]
        n105 = call-poly "Constants Main.vi"("Action"=CD_System_Explorer_lvlib."LibraryFolderName") -> ("Output"=w237:string)  [unwired: 10 in]
        n106 = Build Path(base path=w230, name or relative path=w237) -> (appended path=w239:path)
        n107 = Create Folder(path (use dialog)=w239, error in=w231) -> (created path=w235:path, error out=w236:errorcluster)  [unwired: 1 in, 1 out]
        n108 = To More Specific Class(target class=refnum<class "NIVS_PPLCD Template.lvclass"> refnum ("NIVS_PPLCD Template.lvclass"), reference=w229) -> (error out=w227:errorcluster)  [unwired: 1 in, 1 out]
        n109 = case shown="No Error" w227 {
          tunnel: w236 -> [w245 w250]
          tunnel: w235 -> [w241 w249]
          tunnel: [w244 w248] -> w224
          tunnel: w232 -> [w243 w247]
          tunnel: w229 -> [w242 w246]
          frame No Error {
            n110 = call "System Explorer - Copy PPLTemplates for System Explorer.vi"("CD Name"=w243, "error in (no error)"=w245, "CD Template"=w242, "System Explorer folder"=w241) -> ("error out"=w244:errorcluster)  [unwired: 7 in]
          }
          frame Error {
            n111 = call "System Explorer - Copy Templates for System Explorer.vi"("CD Name"=w247, "error in (no error)"=w250, "CD Template"=w246, "System Explorer folder"=w249) -> ("error out"=w248:errorcluster)  [unwired: 7 in]
          }
        }
        n112 = call <vilib>:"Error Cluster From Error Code.vi"("error in (no error)"=w224, "error message (\"\")"="Current termination point: PC-System Explorer - Create folder and copy templates " ("error message (\"\")"), "error code (0)"=5001) -> ("error out"=w223:errorcluster)  [unwired: 6 in]
      }
      frame "PC-System Explorer - Create extra pages" {
        # "Create a VI for each extra page on the file system."
        n113 = property class="Consolidated_CD"(reference=w255) -> ("Project Name"=w254:string, "Accessors:CD Template"=w253:refnum<class "NIVS_CD Template.lvclass">, "Project Root"=w251:path)  [unwired: 1 in, 2 out]
        n114 = property class="CD Template"(reference=w253) -> ("Accessors:Extra Page Names"=w252:string[])  [unwired: 1 in, 2 out]
        n115 = call-poly "Constants Main.vi"("Action"=CD_System_Explorer_lvlib."LibraryFolderName") -> ("Output"=w263:string)  [unwired: 10 in]
        n116 = call-poly "Constants Main.vi"("Action"=Common."PathToTemplates") -> ("Output"=w259:string)  [unwired: 10 in]
        n117 = String To Path(string=w259) -> (path=w258:path)
        n118 = Build Path(base path=w258, name or relative path=path "Extra Page.vi") -> (appended path=w264:path)
        n119 = Build Path(base path=w251, name or relative path=w263) -> (appended path=w261:path)
        n120 = for "Iterate over all extra pages" {
          tunnel: w252 -> [w269] mode=indexing
          shift-right: [w274] -> w266
          shift-left: w256 -> [w283]
          tunnel: w261 -> [w281]
          tunnel: w264 -> [w282]
          tunnel: w254 -> [w278]
          n121 = Concatenate Strings(w269, ".vi") -> (w284:string)
          n122 = Build Path(base path=w281, name or relative path=w284) -> (appended path=w276:path)
          n123 = Concatenate Strings(w278, ".chm" ("string")) -> (w273:string)
          n124 = call "Copy VI and disconnect it from library.vi"("error in (no error)"=w283, "VI Target Path"=w276, "VI Source Path"=w282) -> ("error out"=w280:errorcluster)  [unwired: 8 in]
          n125 = Concatenate Strings("HTML Help Source/" ("string"), w269, ".html" ("string")) -> (w271:string)
          n126 = call "Set BD string constant value.vi"("error in (no error)"=w280, "Name of string constant"="CD_CHM_FileName", "New String Value"=w273, "Path to VI"=w276) -> ("error out"=w277:errorcluster)  [unwired: 7 in]
          n127 = call "Set BD string constant value.vi"("error in (no error)"=w277, "Name of string constant"="CD_CHM_Section", "New String Value"=w271, "Path to VI"=w276) -> ("error out"=w274:errorcluster)  [unwired: 7 in]
        }
      }
      frame "PC-System Explorer - Create library" {
        # "Create the library for System Explorer components."
        n128 = property class="Consolidated_CD"(reference=w288) -> ("Project Name"=w287:string, "Project Root"=w286:path)  [unwired: 1 in, 2 out]
        n129 = call-poly "Constants Main.vi"("Action"=CD_System_Explorer_lvlib."LibraryFolderName") -> ("Output"=w299:string)  [unwired: 10 in]
        n130 = call-poly "Constants Main.vi"("Action"=CD_System_Explorer_lvlib."LibraryFileName") -> ("Output"=w300:string)  [unwired: 10 in]
        n131 = Format Into String(format string=w300, w287) -> (resulting string=w301:string)  [unwired: 2 in, 1 out]
        n132 = Build Path(base path=w286, name or relative path=w299) -> (appended path=w302:path)
        n133 = Build Path(base path=w302, name or relative path=w301) -> (appended path=w291:path)
        n134 = invoke class="App" method="Library.Create"(error in=w289) -> (error out=w294:errorcluster, "Create Library"=w293:refnum<vi>)  [unwired: 3 in, 2 out]
        n135 = invoke class="Library" method="Save"(reference=w293, error in=w294, "Path"=w291) -> (reference out=w292:refnum<vi>, error out=w290:errorcluster)  [unwired: 1 in, 2 out]
        n136 = Bundle By Name(cluster=w295, "System Explorer Library"=w292) -> (w296:T1)
      }
      frame "PC-System Explorer - Add folders and VIs to library" {
        # "Add virtual folders and all VIs to <CD> System Explorer.lvlib"
        n137 = property class="Consolidated_CD"(reference=w309) -> ("Project Root"=w308:path, "Accessors:CD Template"=w307:refnum<class "NIVS_CD Template.lvclass">)  [unwired: 1 in, 2 out]
        n138 = property class="CD Template"(reference=w307) -> ("Accessors:Extra Page Names"=w306:string[])  [unwired: 1 in, 2 out]
        n139 = call "System Explorer - Add content to System Explorer library.vi"("error in (no error)"=w315, "Extra Page Names"=w306, "Project Root"=w308, "CD Wizard - Internal Data"=w313) -> ("error out"=w314:errorcluster, "Extra Page VIs"=w304:path[], "System Explorer Main VI"=w312:path, "Load Help File VI"=w311:path)  [unwired: 4 in]
        n140 = Build Array (concatenate)(w312, w304) -> (w305:path[])
        n141 = for {
          tunnel: w305 -> [w322] mode=indexing
          tunnel: w311 -> [w321]
          shift-right: [w318] -> w310
          shift-left: w314 -> [w331]
          # "On the diagram of the Main VI and all the Extra Page VIs, replace the stub subVI for Load Help File.vi with the actual new VI."
          n142 = Open VI Reference(vi path=w322, error in (no error)=w331) -> (vi reference=w328:refnum<vi>, error out=w330:errorcluster)  [unwired: 4 in]
          n143 = call <vilib>:"TRef Find Object By Label.vi"("Label"="Load Help File_stub.vi", "Traverse Target"=TRef_TravTarget."BD", "error in (no error)"=w330, "Class Name"="SubVI", "VI Ref"=w328) -> ("error out"=w329:errorcluster, "Found Obj Ref"=w323:refnum<vi>, "dup VI Ref"=w319:refnum<vi>)  [unwired: 3 in, 1 out]
          n144 = invoke class="GObj" method="Replace"(reference=w323, error in=w329, "Path"=w321) -> (error out=w324:errorcluster)  [unwired: 3 in, 5 out]
          n145 = invoke class="VI" method="Save.Instrument"(reference=w319, error in=w324) -> (reference out=w317:refnum<vi>, error out=w320:errorcluster)  [unwired: 4 in, 4 out]
          n146 = Close Reference(reference=w317, error in (no error)=w320) -> (error out=w318:errorcluster)
        }
      }
      frame "PC-Engine - Create folder and copy the RT Template" {
        # "Create a new Engine folder on the file system and copy the RT Driver VI for the chosen custom device."
        n147 = property class="Consolidated_CD"(reference=w335) -> ("Accessors:CD Template"=w332:refnum<class "NIVS_CD Template.lvclass">, "Project Name"=w334:string, "Project Root"=w333:path)  [unwired: 1 in, 2 out]
        n148 = call-dynamic "Create Engine Folder and Copy RT Template.vi"("error in (no error)"=w338, "Project Root"=w333, "Project Name"=w334, "CD Template"=w332) -> ("error out"=w337:errorcluster)  [unwired: 7 in]
      }
      frame "PC-Engine - Create library" {
        # "Create the library for the Engine components."
        n149 = property class="Consolidated_CD"(reference=w342) -> ("Project Name"=w341:string, "Project Root"=w340:path)  [unwired: 1 in, 2 out]
        n150 = call-poly "Constants Main.vi"("Action"=CD_Engine_lvlib."LibraryFolderName") -> ("Output"=w353:string)  [unwired: 10 in]
        n151 = call-poly "Constants Main.vi"("Action"=CD_Engine_lvlib."LibraryFileName") -> ("Output"=w354:string)  [unwired: 10 in]
        n152 = Format Into String(format string=w354, w341) -> (resulting string=w355:string)  [unwired: 2 in, 1 out]
        n153 = Build Path(base path=w340, name or relative path=w353) -> (appended path=w356:path)
        n154 = Build Path(base path=w356, name or relative path=w355) -> (appended path=w344:path)
        n155 = invoke class="App" method="Library.Create"(error in=w343) -> (error out=w348:errorcluster, "Create Library"=w347:refnum<vi>)  [unwired: 3 in, 2 out]
        n156 = invoke class="Library" method="Save"(reference=w347, error in=w348, "Path"=w344) -> (reference out=w345:refnum<vi>, error out=w346:errorcluster)  [unwired: 1 in, 2 out]
        n157 = Bundle By Name(cluster=w350, "Engine Library"=w345) -> (w349:T1)
      }
      frame "PC-Engine - Add virtual folders and VIs to library" {
        # "Add all virtual folders and template VIs to the Engine library"
        n158 = property class="Consolidated_CD"(reference=w362) -> ("Accessors:CD Template"=w360:refnum<class "NIVS_CD Template.lvclass">, "Project Root"=w359:path, "Project Name"=w358:string)  [unwired: 1 in, 2 out]
        n159 = call-dynamic "Add content to Engine library.vi"("Project Name"=w358, "error in (no error)"=w364, "Project Root"=w359, "CD Wizard - Internal Data"=w361, "CD Template"=w360) -> ("error out"=w363:errorcluster)  [unwired: 6 in]
      }
      frame "PC-XML - Create and change file" {
        # "Create the XML file and add it to the project tree"
        n160 = call "XML - Create XML file.vi"("error in (no error)"=w369, "Consolidated_CD"=w366, "CD Wizard - Internal Data"=w367) -> ("error out"=w368:errorcluster)  [unwired: 8 in]
      }
      frame "PC-Help - Copy HTML Files" {
        w385 = "Main"
        w400 = "OPTIONS" ("section")
        # "Write an empty path as default in the \"Base Path\" to enable \"Build CHM.cfg\" to automatically use the realtive path."
        # "Note: We only copy the files here, the get added to the project in the \"Write New Project File\" case since the project doesn't exist (to add the folder to) until that case."
        # "Copy all of the HTML template files to the new help directory, and configure Build CHM file."
        n161 = property class="Consolidated_CD"(reference=w376) -> ("Project Name"=w375:string, "Project Root"=w374:path, "Accessors:CD Template"=w373:refnum<class "NIVS_CD Template.lvclass">)  [unwired: 1 in, 2 out]
        n162 = property class="CD Template"(reference=w373) -> ("Accessors:Extra Page Names"=w372:string[])  [unwired: 1 in, 2 out]
        n163 = Build Path(base path=w374, name or relative path=path "Help") -> (appended path=w384:path)
        n164 = call <vilib>:"Check if File or Folder Exists.vi"("error in (no error)"=w387, "path"=w384) -> ("error out"=w393:errorcluster, "file or folder exists?"=w407:bool, "dup path"=w408:path)  [unwired: 7 in]
        n165 = case shown="True" w407 {
          tunnel: w408 -> [w411 w415]
          tunnel: [w411 w414] -> w379
          tunnel: [w410 w413] -> w394
          tunnel: w393 -> [w410 w412]
          frame False {
          }
          frame True {
            n166 = Delete(path (use dialog)=w415, entire hierarchy (F)=TRUE, error in=w412) -> (deleted path=w414:path, error out=w413:errorcluster)  [unwired: 2 in, 1 out]
          }
        }
        n167 = Build Array (concatenate)(w385, w372) -> (w378:string[])
        n168 = Concatenate Strings("HTML Help Source\\" ("string"), w385, ".htm" ("string")) -> (w389:string)
        n169 = Create Folder(path (use dialog)=w379, error in=w394) -> (created path=w381:path, error out=w380:errorcluster)  [unwired: 1 in, 1 out]
        n170 = call "Call HTML Help Generation Functions Async.vi"("error in (no error)"=w380, "Extra Page Names"=w378, "Destination Base Path"=w381) -> ("error out"=w377:errorcluster)  [unwired: 7 in, 1 out]
        n171 = Build Path(base path=w381, name or relative path="Build CHM.cfg") -> (appended path=w391:path)
        n172 = call <vilib>:"Open Config Data.vi"("error in (no error)"=w377, "configuration file path"=w391) -> ("error out"=w406:errorcluster, "refnum"=w405:T13)  [unwired: 7 in, 1 out]
        n173 = call-poly <vilib>:"Write Key.vi"("section"=w400, "error in (no error)"=w406, "value"=w375, "key"="Title", "refnum"=w405) -> ("error out"=w403:errorcluster, "refnum out"=w402:T13)  [unwired: 4 in, 1 out]
        n174 = call-poly <vilib>:"Write Key.vi"("section"=w400, "error in (no error)"=w403, "value"=w389, "key"="Default Topic", "refnum"=w402) -> ("error out"=w399:errorcluster, "refnum out"=w397:T13)  [unwired: 4 in, 1 out]
        n175 = call-poly <vilib>:"Write Key.vi"("section"=w400, "error in (no error)"=w399, "value"=path "", "key"="Base Path", "refnum"=w397) -> ("error out"=w398:errorcluster, "refnum out"=w396:T13)  [unwired: 4 in, 1 out]
        n176 = call <vilib>:"Close Config Data.vi"("error in (no error)"=w398, "refnum"=w396) -> ("error out"=w386:errorcluster)  [unwired: 8 in, 1 out]
      }
      frame "Project - Read project file content" {
        w428 = -1  # Read all lines
        w427 = T12."open"  # operation
        w426 = enum16{"read/write", "read-only", "write-only"}."read-only"  # access
        # "Open the project file and read the complete content."
        n177 = call-poly "Constants Main.vi"("Action"=Common."ProjectTemplatePathAndName") -> ("Output"=w419:string)  [unwired: 10 in]
        n178 = String To Path(string=w419) -> (path=w420:path)
        n179 = Open/Create/Replace File(file path (use dialog)=w420, error in=w417, operation (0:open)=w427, access (0:read/write)=w426) -> (refnum out=w424:refnum<file>, error out=w425:errorcluster)  [unwired: 3 out]
        n180 = Read from Text File(file (use dialog)=w424, count=w428, error in=w425) -> (refnum out=w418:refnum<file>, text=w422:string[], error out=w423:errorcluster)  [unwired: 2 out]
        n181 = Close File(refnum=w418) -> ()  [unwired: 1 in, 2 out]
      }
      frame "Project - Edit Utility section" {
        # "Edit the entries for the utility folder. Also added CHM pre build action entries"
        n182 = call-poly "Constants Main.vi"("Action"=Utility_folder."Utility.FolderName") -> ("Output"=w435:string)  [unwired: 10 in]
        n183 = call-poly "Constants Main.vi"("Action"=Utility_folder."Utility.Copy .llb to NI VeriStand dir.FileName") -> ("Output"=w436:string)  [unwired: 10 in]
        n184 = call-poly "Constants Main.vi"("Action"=Utility_folder."Utility.LLB Pre Build.FilePathAndName") -> ("Output"=w433:string)  [unwired: 10 in]
        n185 = String To Path(string=w433) -> (path=w432:path)
        n186 = Strip Path(path=w432) -> (name=w431:string)  [unwired: 1 out]
        n187 = for "For Iterate over each line and change the placeholders for the Utility entries." {
          tunnel: w441 -> [w453] mode=indexing
          shift-right: [w449] -> w439
          shift-left: w430 -> [w451]
          tunnel: [w447] -> w440 mode=indexing
          tunnel: w436 -> [w452]
          tunnel: w435 -> [w450]
          tunnel: w431 -> [w443]
          w445 = TRUE  # ignore case?
          w446 = TRUE  # replace all?
          w456 = "%CopyLLBtoNIVSFileName%"  # search
          w458 = "%UtilityFolderName%"  # search
          # "CHM Build VI as pre-build action"
          # "Copy .LLB to NI VeriStand dir.vi"
          # "Utility"
          n188 = Search and Replace String(replace all?=w446, case sensitive?=w445, input string=w453, search string=w458, replace string=w450, error in=w451) -> (result string=w457:string, error out=w455:errorcluster)  [unwired: 2 in, 2 out]
          n189 = Search and Replace String(replace all?=w446, case sensitive?=w445, input string=w457, search string=w456, replace string=w452, error in=w455) -> (result string=w448:string, error out=w454:errorcluster)  [unwired: 2 in, 2 out]
          n190 = Search and Replace String(replace all?=w446, case sensitive?=w445, input string=w448, search string="%CHMPreBuild%" ("result string"), replace string=w443, error in=w454) -> (result string=w447:string, error out=w449:errorcluster)  [unwired: 2 in, 2 out]
        }
      }
      frame "Project - Edit XML section" {
        # "Edit the Name and Path for the XML file."
        n191 = property class="Consolidated_CD"(reference=w461) -> ("Project Name"=w460:string, "Accessors:CD Template"=w459:refnum<class "NIVS_CD Template.lvclass">)  [unwired: 1 in, 2 out]
        n192 = call "XML - Get XML file name.vi"("CD Template"=w459, "CD Name"=w460) -> ("XML file name"=w463:string)  [unwired: 9 in]
        n193 = for "Iterate over each line and change the placeholder for the XML file name." {
          tunnel: w466 -> [w474] mode=indexing
          shift-right: [w473] -> w467
          shift-left: w462 -> [w469]
          tunnel: [w472] -> w465 mode=indexing
          tunnel: w463 -> [w468]
          w470 = TRUE  # ignore case?
          w471 = TRUE  # replace all?
          w475 = "%XMLCustomDeviceFileName%"  # search
          n194 = Search and Replace String(replace all?=w471, case sensitive?=w470, input string=w474, search string=w475, replace string=w468, error in=w469) -> (result string=w472:string, error out=w473:errorcluster)  [unwired: 2 in, 2 out]
        }
      }
      frame "Project - Edit Engine Library section" {
        # "Edit the entries for the Engine Library (Library name and folder name)"
        n195 = property class="Consolidated_CD"(reference=w477) -> ("Project Name"=w476:string)  [unwired: 1 in, 2 out]
        n196 = call "Change Engine Library Placeholders in project.vi"("error in (no error)"=w481, "Project Name"=w476, "Project file content in"=w478) -> ("error out"=w480:errorcluster, "Project file content out"=w482:string[])  [unwired: 7 in]
      }
      frame "Project - Edit Shared Library section" {
        # "Edit the entries for the Shared Library (Library name and folder name)"
        n197 = property class="Consolidated_CD"(reference=w484) -> ("Project Name"=w483:string)  [unwired: 1 in, 2 out]
        n198 = call-poly "Constants Main.vi"("Action"=CD_Shared_lvlib."LibraryFileName") -> ("Output"=w492:string)  [unwired: 10 in]
        n199 = call-poly "Constants Main.vi"("Action"=CD_Shared_lvlib."LibraryFolderName") -> ("Output"=w488:string)  [unwired: 10 in]
        n200 = call-poly "Constants Main.vi"("Action"=CD_Shared_lvlib."Shared.FolderName") -> ("Output"=w487:string)  [unwired: 10 in]
        n201 = Format Into String(format string=w492, w483) -> (resulting string=w489:string)  [unwired: 2 in, 1 out]
        n202 = for "Iterate over each line and change the placeholder for the Shared Library file and folder name." {
          tunnel: w490 -> [w511] mode=indexing
          shift-right: [w504] -> w495
          shift-left: w485 -> [w510]
          tunnel: [w505] -> w496 mode=indexing
          tunnel: w489 -> [w499]
          tunnel: w488 -> [w498]
          tunnel: w487 -> [w497]
          w502 = "%SharedLibrarySubfolderName%"  # search
          w508 = "%SharedLibraryFolderName%"  # search
          w500 = TRUE  # ignore case?
          w501 = TRUE  # replace all?
          w512 = "%SharedLibraryFileName%"  # search
          # "Shared"
          # "Shared"
          # "<CD> Shared.lvlib"
          n203 = Search and Replace String(replace all?=w501, case sensitive?=w500, input string=w511, search string=w512, replace string=w499, error in=w510) -> (result string=w509:string, error out=w507:errorcluster)  [unwired: 2 in, 2 out]
          n204 = Search and Replace String(replace all?=w501, case sensitive?=w500, input string=w509, search string=w508, replace string=w498, error in=w507) -> (result string=w506:string, error out=w503:errorcluster)  [unwired: 2 in, 2 out]
          n205 = Search and Replace String(replace all?=w501, case sensitive?=w500, input string=w506, search string=w502, replace string=w497, error in=w503) -> (result string=w505:string, error out=w504:errorcluster)  [unwired: 2 in, 2 out]
        }
      }
      frame "Project - Edit System Explorer Library section" {
        # "Edit the entries for the System Explorer Library (Library name and folder name)"
        n206 = property class="Consolidated_CD"(reference=w514) -> ("Project Name"=w513:string)  [unwired: 1 in, 2 out]
        n207 = call-poly "Constants Main.vi"("Action"=CD_System_Explorer_lvlib."LibraryFileName") -> ("Output"=w521:string)  [unwired: 10 in]
        n208 = Format Into String(format string=w521, w513) -> (resulting string=w524:string)  [unwired: 2 in, 1 out]
        n209 = call-poly "Constants Main.vi"("Action"=CD_System_Explorer_lvlib."System Explorer.FolderName") -> ("Output"=w526:string)  [unwired: 10 in]
        n210 = call-poly "Constants Main.vi"("Action"=CD_System_Explorer_lvlib."LibraryFolderName") -> ("Output"=w525:string)  [unwired: 10 in]
        n211 = for "Iterate over each line and change the placeholder for the System Explorer Library file and folder name." {
          tunnel: w517 -> [w541] mode=indexing
          shift-right: [w533] -> w519
          shift-left: w515 -> [w540]
          tunnel: [w534] -> w518 mode=indexing
          tunnel: w524 -> [w529]
          tunnel: w525 -> [w528]
          tunnel: w526 -> [w527]
          w530 = "%SystemExplorerSubfolderName%"  # search
          w538 = "%SystemExplorerLibraryFolderName%"  # search
          w532 = TRUE  # ignore case?
          w531 = TRUE  # replace all?
          w542 = "%SystemExplorerLibraryFileName%"  # search
          n212 = Search and Replace String(replace all?=w531, case sensitive?=w532, input string=w541, search string=w542, replace string=w529, error in=w540) -> (result string=w539:string, error out=w537:errorcluster)  [unwired: 2 in, 2 out]
          n213 = Search and Replace String(replace all?=w531, case sensitive?=w532, input string=w539, search string=w538, replace string=w528, error in=w537) -> (result string=w535:string, error out=w536:errorcluster)  [unwired: 2 in, 2 out]
          n214 = Search and Replace String(replace all?=w531, case sensitive?=w532, input string=w535, search string=w530, replace string=w527, error in=w536) -> (result string=w534:string, error out=w533:errorcluster)  [unwired: 2 in, 2 out]
        }
      }
      frame "Project - Edit Custom Device Name" {
        # "Edit the Custom Device name"
        n215 = property class="Consolidated_CD"(reference=w544) -> ("Project Name"=w543:string)  [unwired: 1 in, 2 out]
        n216 = for "Iterate over each line and change the placeholder for the Custom Device name." {
          tunnel: w546 -> [w556] mode=indexing
          shift-right: [w551] -> w548
          shift-left: w549 -> [w552]
          tunnel: [w555] -> w547 mode=indexing
          tunnel: w543 -> [w550]
          w553 = TRUE  # ignore case?
          w554 = TRUE  # replace all?
          w557 = "%CustomDeviceName%"  # search
          # "<CD>"
          n217 = Search and Replace String(replace all?=w554, case sensitive?=w553, input string=w556, search string=w557, replace string=w550, error in=w552) -> (result string=w555:string, error out=w551:errorcluster)  [unwired: 2 in, 2 out]
        }
      }
      frame "Project - Edit System Explorer LLB Name" {
        # "Edit the name for the System Explorer LLB."
        n218 = property class="Consolidated_CD"(reference=w559) -> ("Project Name"=w558:string)  [unwired: 1 in, 2 out]
        n219 = call-poly "Constants Main.vi"("Action"=Build_Spec_System_Explorer."Destinations.LLBFileName") -> ("Output"=w566:string)  [unwired: 10 in]
        n220 = Format Into String(format string=w566, w558) -> (resulting string=w563:string)  [unwired: 2 in, 1 out]
        n221 = for "Iterate over each line and change the placeholder for the System Explorer LLB." {
          tunnel: w563 -> [w573]
          tunnel: w562 -> [w571] mode=indexing
          tunnel: [w570] -> w561 mode=indexing
          shift-right: [w569] -> w567
          shift-left: w560 -> [w572]
          w568 = "%SystemExplorerLLBFileName%"  # search
          w574 = TRUE  # ignore case?
          w575 = TRUE  # replace all?
          # "<CD> Configuration.llb"
          n222 = Search and Replace String(replace all?=w575, case sensitive?=w574, input string=w571, search string=w568, replace string=w573, error in=w572) -> (result string=w570:string, error out=w569:errorcluster)  [unwired: 1 in, 3 out]
        }
      }
      frame "Project - Edit Engine LLB OS dependent file name" {
        n223 = property class="Consolidated_CD"(reference=w577) -> ("Project Name"=w576:string)  [unwired: 1 in, 2 out]
        n224 = call-poly "Constants Main.vi"("Action"=Build_Spec_Engine."Destinations.LLBLinux64FileName") -> ("Output"=w587:string)  [unwired: 10 in]
        n225 = call-poly "Constants Main.vi"("Action"=Build_Spec_Engine."Destinations.LLBLinuxARMFileName") -> ("Output"=w588:string)  [unwired: 10 in]
        n226 = call-poly "Constants Main.vi"("Action"=Build_Spec_Engine."Destinations.LLBPharlapFileName") -> ("Output"=w593:string)  [unwired: 10 in]
        n227 = call-poly "Constants Main.vi"("Action"=Build_Spec_Engine."Destinations.LLBWindowsFileName") -> ("Output"=w598:string)  [unwired: 10 in]
        n228 = call-poly "Constants Main.vi"("Action"=Build_Spec_Engine."Destinations.LLBVxWorksFileName") -> ("Output"=w594:string)  [unwired: 10 in]
        n229 = Format Into String(format string=w587, w576) -> (resulting string=w581:string)  [unwired: 2 in, 1 out]
        n230 = Format Into String(format string=w588, w576) -> (resulting string=w582:string)  [unwired: 2 in, 1 out]
        n231 = Format Into String(format string=w598, w576) -> (resulting string=w585:string)  [unwired: 2 in, 1 out]
        n232 = Format Into String(format string=w594, w576) -> (resulting string=w584:string)  [unwired: 2 in, 1 out]
        n233 = Format Into String(format string=w593, w576) -> (resulting string=w583:string)  [unwired: 2 in, 1 out]
        n234 = Build Array(w585, w584, w583, w582, w581) -> (w580:string[])
        n235 = for {
          shift-right: [w603] -> w590
          shift-left: w578 -> [w604]
          tunnel: w591 -> [w600] mode=indexing
          tunnel: w580 -> [w601]
          tunnel: [w599] -> w579 mode=indexing
          n236 = for {
            shift-right: [w612] -> w603
            shift-left: w604 -> [w611]
            shift-right: [w608] -> w599
            shift-left: w600 -> [w607]
            tunnel: string[] ["%EngineLLBWindowsFileName%", "%EngineLLBVxWorksFileName%", "%EngineLLBPharlapFileName%", "%EngineLLBLinuxARMFileName%", "%EngineLLBLinux64FileName%"] -> [w606] mode=indexing
            tunnel: w601 -> [w605] mode=indexing
            w609 = TRUE  # ignore case?
            w610 = TRUE  # replace all?
            n237 = Search and Replace String(replace all?=w610, case sensitive?=w609, input string=w607, search string=w606, replace string=w605, error in=w611) -> (result string=w608:string, error out=w612:errorcluster)  [unwired: 1 in, 3 out]
          }
        }
      }
      frame "Project - Copy Configuration file" {
        n238 = property class="Consolidated_CD"(reference=w620) -> ("Project Name"=w622:string, "Project Root"=w621:path)  [unwired: 1 in, 2 out]
        n239 = call-poly "Constants Main.vi"("Action"=Common."ProjectConfigurationName") -> ("Output"=w623:string)  [unwired: 10 in]
        n240 = Format Into String(format string=w623, w622) -> (resulting string=w625:string)  [unwired: 2 in, 1 out]
        n241 = call-poly "Constants Main.vi"("Action"=Common."PathToConfigurationFile") -> ("Output"=w618:string)  [unwired: 10 in]
        n242 = Build Path(base path=w621, name or relative path=w625) -> (appended path=w616:path)
        n243 = String To Path(string=w618) -> (path=w617:path)
        n244 = Copy(8:w615, 9:FALSE ("overwrite (F)"), 10:w616, 11:w617) -> (0:w614:errorcluster)  [unwired: 1 in, 2 out]
      }
      frame "Project - Write new project file" {
        # "Create new file and write the project file content into it."
        n245 = property class="Consolidated_CD"(reference=w630) -> ("Project Name"=w629:string, "Project Root"=w628:path)  [unwired: 1 in, 2 out]
        n246 = call-poly "Constants Main.vi"("Action"=Common."ProjectName") -> ("Output"=w654:string)  [unwired: 10 in]
        n247 = Format Into String(format string=w654, w629) -> (resulting string=w665:string)  [unwired: 2 in, 1 out]
        n248 = Build Path(base path=w628, name or relative path=w665) -> (appended path=w660:path)
        n249 = Open/Create/Replace File(file path (use dialog)=w660, error in=w631, operation (0:open)=T12."replace or create") -> (refnum out=w662:refnum<file>, error out=w661:errorcluster)  [unwired: 3 in, 1 out]
        n250 = Write to Text File(file (use dialog)=w662, text=w657, error in=w661) -> (refnum out=w659:refnum<file>, error out=w658:errorcluster)  [unwired: 2 out]
        n251 = Close File(refnum=w659, error in=w658) -> (path=w655:path, error out=w653:errorcluster)
        n252 = invoke class="App" method="Project.Open"(error in=w653, "Path"=w655) -> (error out=w648:errorcluster, "Project:Open"=w647:refnum<vi>)  [unwired: 2 in, 2 out]
        n253 = Build Path(base path=w628, name or relative path=path "Help") -> (appended path=w641:path)
        n254 = property class="Project"(reference=w647, error in=w648) -> (reference out=w646:refnum<vi>, error out=w644:errorcluster, "My Computer"=w645:refnum<vi>)
        n255 = invoke class="TargetItem" method="AddItem"(reference=w645, error in=w644, "Name"="Placeholder", "Path"=path "", "Type"="Folder") -> (reference out=w634:refnum<vi>, error out=w651:errorcluster, "AddItem"=w650:refnum<vi>)  [unwired: 1 in, 3 out]
        n256 = invoke class="ProjectItem" method="Convert to Auto-populating Folder"(reference=w650, error in=w651, "Path"=w641) -> (reference out=w636:refnum<vi>, error out=w632:errorcluster)  [unwired: 1 in, 2 out]
        n257 = Close Reference(reference=w636) -> (error out=w635:errorcluster)  [unwired: 1 in]
        n258 = invoke class="Project" method="Open Window"(reference=w646, error in=w632) -> (reference out=w633:refnum<vi>, error out=w637:errorcluster)  [unwired: 1 in, 1 out]
        n259 = Close Reference(reference=w634, error in (no error)=w635) -> ()  [unwired: 1 out]
        n260 = invoke class="Project" method="Save"(reference=w633, error in=w637) -> (reference out=w639:refnum<vi>, error out=w640:errorcluster)  [unwired: 2 in, 2 out]
        n261 = Close Reference(reference=w639, error in (no error)=w640) -> (error out=w638:errorcluster)
      }
    }
  }
  "error out" <- w6
  n262 = disable-structure shown="Disabled" {
    frame Disabled {
      n263 = call <vilib>:"Error Cluster From Error Code.vi"("error message (\"\")"="Generic error" ("error message (\"\")"), "error code (0)"=5001) -> ("error in (no error)"=w668:errorcluster)  [unwired: 6 in, 1 out]
    }
    frame Enabled {
    }
  }
